vi "testParseIDLFile.vi"(8 "error in (no error)":errorcluster) -> (0 "error out":errorcluster)   [LabVIEW 2018]
uses:
  SALTypeGenerator/IDLFile/IDLFile.lvclass
  SALTypeGenerator/IDLFile/IDLFile.lvclass/IDLFile.ctl
  SALTypeGenerator/Module/Module.lvclass/Module.ctl
  <vilib>/addons/_JKI Toolkits/Caraya/classes/Assert/Assert Equal Value_Variant.vi
  SALTypeGenerator/Module/Module.lvclass
  SALTypeGenerator/Topic/Topic.lvclass
  SALTypeGenerator/Enumeration/Enumeration.lvclass
  <vilib>/addons/_JKI Toolkits/Caraya/classes/Test/Test.lvclass
  <vilib>/addons/_JKI Toolkits/Caraya/classes/Assert/Assert.lvclass
  SALTypeGenerator/Element/Element.lvclass
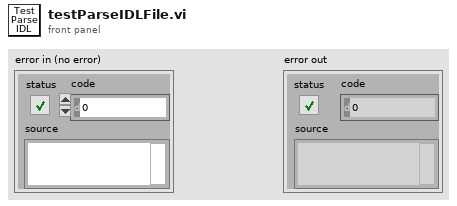
[diagram p1: front panel]
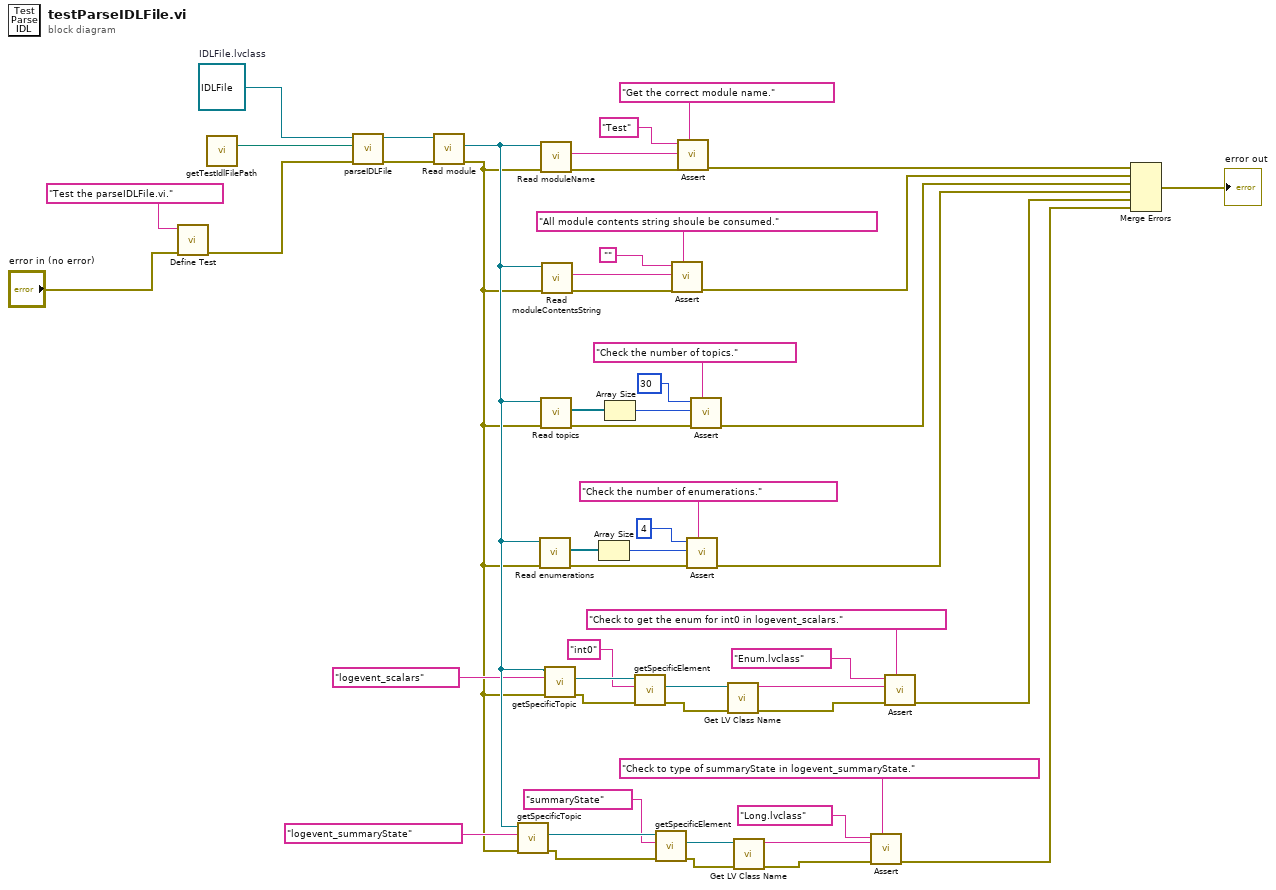
[diagram p0: block diagram]
diagram:
  w53 = refnum<class "IDLFile.lvclass"> refnum  # IDLFile.lvclass
  n1 = call <vilib>:"Define Test.vi"("error in (no error)"="error in (no error)", "Label (VI Title)"="Test the parseIDLFile.vi.") -> ("error out"=w48:errorcluster)  [unwired: 9 in]
  n2 = call "getTestIdlFilePath.vi"() -> ("testIdlPath"=w54:path)  [unwired: 11 in]
  n3 = call "parseIDLFile.vi"("error in (no error)"=w48, "idlFilepath"=w54, "IDLFile in"=w53) -> ("error out"=w52:errorcluster, "IDLFile out"=w51:refnum<class "IDLFile.lvclass">)  [unwired: 7 in]
  n4 = call "Read module.vi"("error in (no error)"=w52, "IDLFile in"=w51) -> ("error out"=w11:errorcluster, "Module.lvclass"=w13:refnum<class "Module.lvclass">)  [unwired: 7 in, 1 out]
  n5 = call "getSpecificTopic.vi"("error in (no error)"=w11, "nameTopic"="logevent_summaryState" ("topicName"), "Module in"=w13) -> ("error out"=w9:errorcluster, "Topic.lvclass"=w10:refnum<class "Topic.lvclass">)  [unwired: 6 in, 1 out]
  n6 = call "Read enumerations.vi"("error in (no error)"=w11, "Module in"=w13) -> ("error out"=w28:errorcluster, "enumerations"=w30:refnum<class "Enumeration.lvclass">[])  [unwired: 7 in, 1 out]
  n7 = call "Read moduleName.vi"("error in (no error)"=w11, "Module in"=w13) -> ("error out"=w47:errorcluster, "moduleName"=w46:string)  [unwired: 7 in, 1 out]
  n8 = call "Read topics.vi"("error in (no error)"=w11, "Module in"=w13) -> ("error out"=w34:errorcluster, "topics"=w36:refnum<class "Topic.lvclass">[])  [unwired: 7 in, 1 out]
  n9 = call "Read moduleContentsString.vi"("error in (no error)"=w11, "Module in"=w13) -> ("error out"=w43:errorcluster, "moduleContentsString"=w42:string)  [unwired: 7 in, 1 out]
  n10 = call "getSpecificTopic.vi"("error in (no error)"=w11, "nameTopic"="logevent_scalars" ("topicName"), "Module in"=w13) -> ("error out"=w3:errorcluster, "Topic.lvclass"=w5:refnum<class "Topic.lvclass">)  [unwired: 6 in, 1 out]
  n11 = Array Size(array=w30) -> (size(s)=w29:i32)
  n12 = Array Size(array=w36) -> (size(s)=w35:i32)
  n13 = call "getSpecificElement.vi"("error in (no error)"=w3, "nameElem"="int0", "Topic in"=w5) -> ("error out"=w1:errorcluster, "Element.lvclass"=w2:refnum<class "Element.lvclass">)  [unwired: 6 in, 1 out]
  n14 = call "getSpecificElement.vi"("error in (no error)"=w9, "nameElem"="summaryState" ("topicName"), "Topic in"=w10) -> ("error out"=w6:errorcluster, "Element.lvclass"=w7:refnum<class "Element.lvclass">)  [unwired: 6 in, 1 out]
  n15 = call-poly <vilib>:"Assert.vi"("Label"="All module contents string shoule be consumed.", "error in (no error)"=w43, "Y"=w42, "X"="") -> ("error out"=w38:errorcluster)  [unwired: 7 in]
  n16 = call-poly <vilib>:"Assert.vi"("Label"="Get the correct module name.", "error in (no error)"=w47, "Y"=w46, "X"="Test") -> ("error out"=w39:errorcluster)  [unwired: 7 in]
  n17 = call-poly <vilib>:"Assert.vi"("Label"="Check the number of enumerations.", "error in (no error)"=w28, "Y"=w29, "X"=4) -> ("error out"=w25:errorcluster)  [unwired: 7 in]
  n18 = call-poly <vilib>:"Assert.vi"("Label"="Check the number of topics.", "error in (no error)"=w34, "Y"=w35, "X"=30) -> ("error out"=w31:errorcluster)  [unwired: 7 in]
  n19 = call <vilib>:"Get LV Class Name.vi"("error in (no error)"=w1, "object"=w2) -> ("error out"=w22:errorcluster, "class name"=w24:string)  [unwired: 8 in]
  n20 = call <vilib>:"Get LV Class Name.vi"("error in (no error)"=w6, "object"=w7) -> ("error out"=w18:errorcluster, "class name"=w19:string)  [unwired: 8 in]
  n21 = call-poly <vilib>:"Assert.vi"("Label"="Check to type of summaryState in logevent_summaryState.", "error in (no error)"=w18, "Y"=w19, "X"="Long.lvclass") -> ("error out"=w15:errorcluster)  [unwired: 7 in]
  n22 = call-poly <vilib>:"Assert.vi"("Label"="Check to get the enum for int0 in logevent_scalars.", "error in (no error)"=w22, "Y"=w24, "X"="Enum.lvclass") -> ("error out"=w20:errorcluster)  [unwired: 7 in]
  n23 = Merge Errors(w39, w38, w31, w25, w20, w15) -> (→"error out":errorcluster)
